vi "Delete Template Files.vi"(8 "error in (no error)":errorcluster, 11 "LVClassLibrary in":refnum<vi>) -> (0 "error out":errorcluster, 3 "LVClassLibrary out":refnum<vi>)   [LabVIEW 2019, in "gRPC Scripting Tools.lvlib"]
uses:
  gRPC Scripting Tools.lvlib
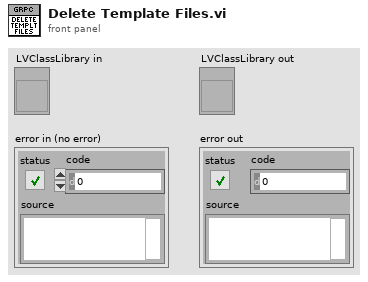
[diagram p1: front panel]
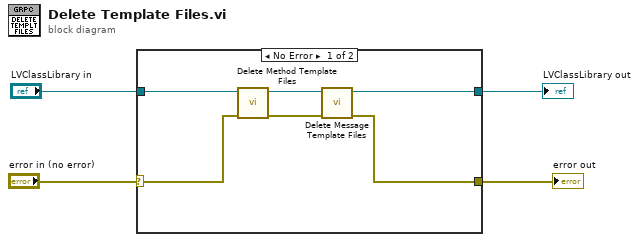
[diagram p0: block diagram]
diagram:
  n1 = case shown="No Error" "error in (no error)" {
    selector: "error in (no error)" -> [w5 w11]
    tunnel: [w10 w12] -> w4
    tunnel: [w9 w11] -> w3
    tunnel: "LVClassLibrary in" -> [w6 w12]
    frame No Error {
      n2 = call "Delete Method Template Files.vi"("error in (no error)"=w5, "LVClassLibrary in"=w6) -> ("error out"=w7:errorcluster, "LVClassLibrary out"=w8:refnum<vi>)  [unwired: 8 in]
      n3 = call "Delete Message Template Files.vi"("error in (no error)"=w7, "LVClassLibrary in"=w8) -> ("error out"=w9:errorcluster, "LVClassLibrary out"=w10:refnum<vi>)  [unwired: 8 in]
    }
    frame Error {
    }
  }
  "LVClassLibrary out" <- w4
  "error out" <- w3
